vi "Adjust Controls to Run Level.vi"(8 "error in (no error)":errorcluster, 9 "Level 30 Controls":refnum<vi>[](array[refnum]), 10 "Level 20 Controls":refnum<vi>[](array[refnum]), 11 "Level 10 Controls":refnum<vi>[](array[refnum])) -> (0 "error out":errorcluster)   [LabVIEW 2019]
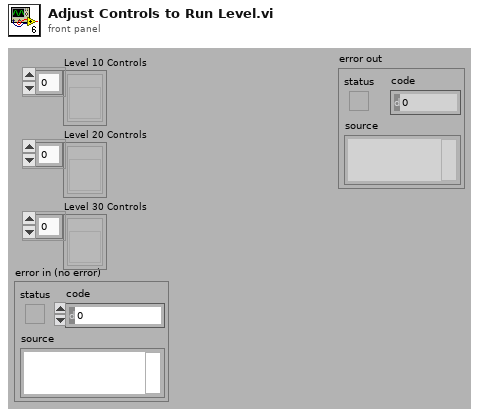
[diagram p1: front panel]
types:
  T1 = enum8{"Enabled", "Disabled", "Disabled and Grayed Out"}
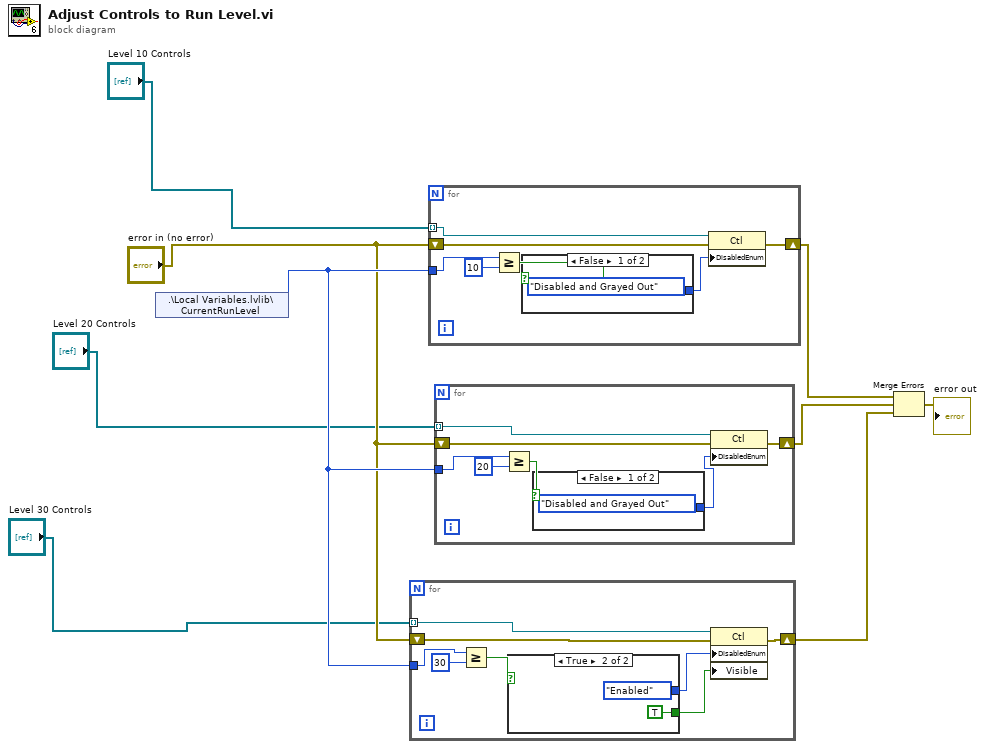
[diagram p0: block diagram]
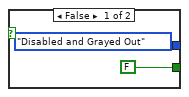
[diagram p2: hidden frame]
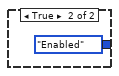
[diagram p3: hidden frame]
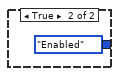
[diagram p4: hidden frame]
diagram:
  n1 = shared-variable ".\\Local Variables.lvlib\\CurrentRunLevel"() -> (w9:i32)  [unwired: 1 in, 1 out]
  n2 = for {
    tunnel: "Level 30 Controls" -> [w15] mode=indexing
    tunnel: w9 -> [w17]
    shift-right: [w13] -> w5
    shift-left: "error in (no error)" -> [w14]
    n3 = Greater Or Equal?(x=w17, y=30) -> (x >= y?=w12:bool)
    n4 = case shown="True" w12 {
      tunnel: [T1."Disabled and Grayed Out" ("Disabled") T1."Enabled" ("Disabled")] -> w11
      tunnel: [FALSE TRUE] -> w10
      frame False {
      }
      frame True {
      }
    }
    n5 = property class="Ctl"(reference=w15, error in=w14, "DisabledEnum"=w11, "Visible"=w10) -> (error out=w13:errorcluster)  [unwired: 1 out]
  }
  n6 = for {
    tunnel: "Level 10 Controls" -> [w26] mode=indexing
    tunnel: w9 -> [w28]
    shift-right: [w24] -> w7
    shift-left: "error in (no error)" -> [w25]
    n7 = Greater Or Equal?(x=w28, y=10) -> (x >= y?=w23:bool)
    n8 = case shown="False" w23 {
      tunnel: [T1."Disabled and Grayed Out" ("Disabled") T1."Enabled" ("Disabled")] -> w22
      frame False {
      }
      frame True {
      }
    }
    n9 = property class="Ctl"(reference=w26, error in=w25, "DisabledEnum"=w22) -> (error out=w24:errorcluster)  [unwired: 1 out]
  }
  n10 = for {
    tunnel: "Level 20 Controls" -> [w35] mode=indexing
    tunnel: w9 -> [w37]
    shift-right: [w33] -> w6
    shift-left: "error in (no error)" -> [w34]
    n11 = Greater Or Equal?(x=w37, y=20) -> (x >= y?=w32:bool)
    n12 = case shown="False" w32 {
      tunnel: [T1."Disabled and Grayed Out" ("Disabled") T1."Enabled" ("Disabled")] -> w31
      frame False {
      }
      frame True {
      }
    }
    n13 = property class="Ctl"(reference=w35, error in=w34, "DisabledEnum"=w31) -> (error out=w33:errorcluster)  [unwired: 1 out]
  }
  n14 = Merge Errors(w7, w6, w5) -> (→"error out":errorcluster)
